vi "Test_MergeErrorsPublication_ErrorArray_1stErrorMerged.vi"(8 "error in (no error)":errorcluster, 11 "TestCase in":refnum<class "TestPublicationPolicy.lvclass">) -> (0 "error out":errorcluster, 3 "TestCase out":refnum<class "TestPublicationPolicy.lvclass">)   [LabVIEW 2020, in "TestPublicationPolicy.lvclass"]
uses:
  TestPublicationPolicy.lvclass
  TestPublicationPolicy.lvclass/TestPublicationPolicy.ctl
  Source/IMediator/MutexedPublishRequest/MutexedPublishRequest.lvclass
  Source/IMediator/IPublicationPolicy/IPublicationPolicy.lvclass
  Source/PublicationPolicy/MergeErrorsPublication/MergeErrorsPublication.lvclass
  modules/composed-transport/Source/Concrete/NotifierTransport/NotifierTransport.lvclass
  C:/Git/mva-core/Source/IMediator/IPublicationPolicy/IPublicationPolicy.lvclass
  C:/Git/mva-core/Source/PublicationPolicy/MergeErrorsPublication/MergeErrorsPublication.lvclass
  C:/Git/mva-core/modules/composed-transport/Source/ITransport/ITransport.lvclass
  C:/Git/mva-core/modules/composed-transport/Source/Concrete/NotifierTransport/NotifierTransport.lvclass
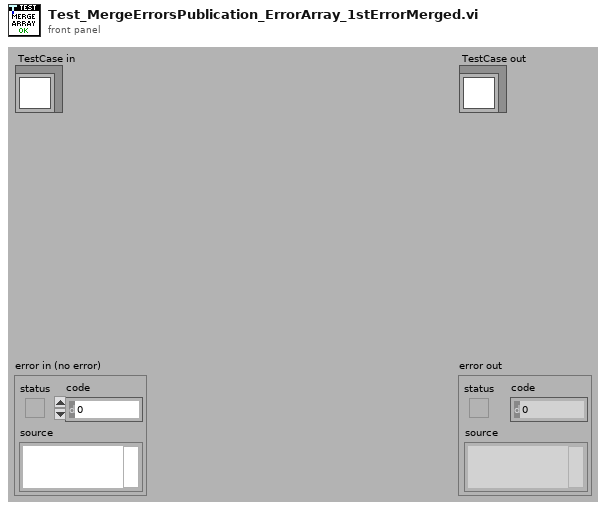
[diagram p1: front panel]
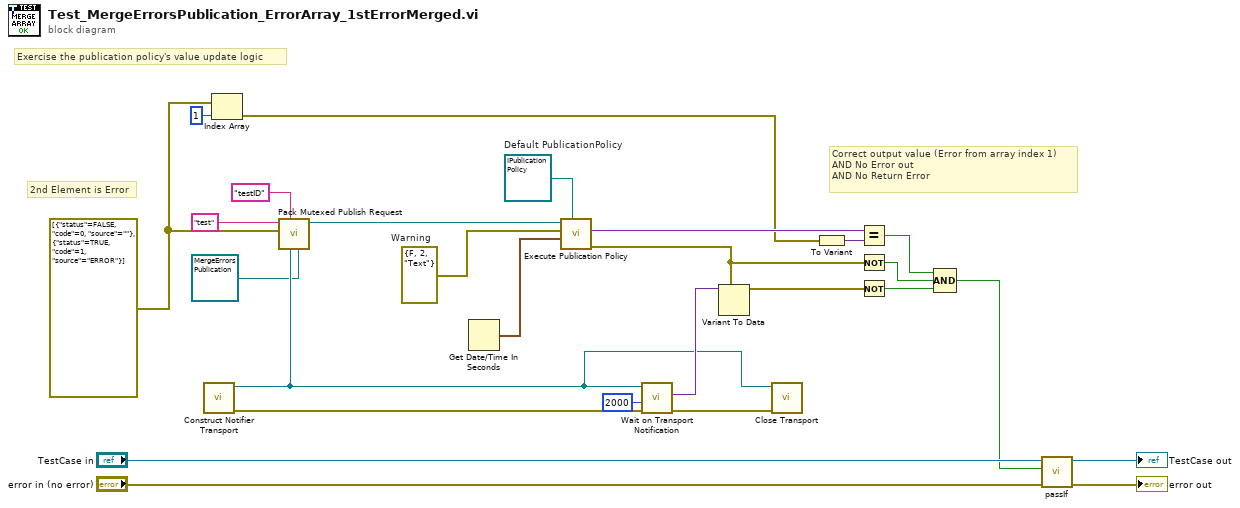
[diagram p0: block diagram]
diagram:
  w6 = errorcluster[] [{"status"=FALSE, "code"=0, "source"=""}, {"status"=TRUE, "code"=1, "source"="ERROR"}] ("error constant")
  w21 = refnum<class "IPublicationPolicy.lvclass"> refnum  # Default PublicationPolicy
  w7 = errorcluster {"status"=FALSE, "code"=2, "source"="Text"}  # Warning
  # "2nd Element is Error"
  # "Correct output value (Error from array index 1)\nAND No Error out\nAND No Return Error"
  # "Exercise the publication policy's value update logic"
  n1 = call "Construct Notifier Transport.vi"() -> ("error out"=w18:errorcluster, "NotifierTransport"=w3:refnum<class "NotifierTransport.lvclass">)  [unwired: 10 in]
  n2 = Index Array(array=w6, index=1) -> (element=w4:errorcluster)
  n3 = call "Pack Mutexed Publish Request.vi"("PublicationPolicy"=refnum<class "MergeErrorsPublication.lvclass"> refnum ("PublicationPolicy.lvlib:MergeErrorsPublication.lvclass"), "Return Error Transport"=w3, "Publisher ID"="testID", "Datum Value or Type"=w6, "Datum Name"="test") -> ("MutexedPublishRequest Out"=w22:refnum<class "MutexedPublishRequest.lvclass">)  [unwired: 5 in, 1 out]
  n4 = Get Date/Time In Seconds() -> (seconds since 1Jan1904=w23:timestamp)
  n5 = call-dynamic "Execute Publication Policy.vi"("Default PublicationPolicy"=w21, "Last Publish Time"=w23, "Last Published Value"=w7, "MutexedPublishRequest"=w22) -> ("error out (Reject Publication)"=w10:errorcluster, "Value to Publish"=w15:variant)  [unwired: 5 in, 1 out]
  n6 = call "Wait on Transport Notification.vi"("error in (no error)"=w18, "Timeout In ms (-1)"=2000, "NotifierTransport"=w3) -> ("error out"=w2:errorcluster, "Data"=w16:variant)  [unwired: 6 in, 1 out]
  n7 = Variant To Data(type=w10, Variant=w16) -> (data=w13:errorcluster)  [unwired: 1 in, 1 out]
  n8 = call-dynamic "Close Transport.vi"("error in (no error)"=w2, "NotifierTransport"=w3) -> ()  [unwired: 9 in, 1 out]
  n9 = To Variant(anything=w4) -> (Variant=w14:variant)
  n10 = Equal?(x=w15, y=w14) -> (x = y?=w12:bool)
  n11 = Not(x=w10) -> (.not. x?=w9:bool)
  n12 = Not(x=w13) -> (.not. x?=w11:bool)
  n13 = Compound Arithmetic op=AND(w12, w9, w11) -> (w8:bool)
  n14 = call-dynamic "passIf.vi"("error in (no error)"="error in (no error)", "pass"=w8, "TestCase in"="TestCase in") -> ("error out"=→"error out":errorcluster, "TestCase out"=→"TestCase out":refnum<class "TestPublicationPolicy.lvclass">)  [unwired: 7 in]
